vi "Load Clusters from BIN FIles_Core.vi"() -> (1 "System settings":T1={"CONFIG Folder - Relative Path "=path "", "FIFO Depth (# of elements)"=0, "Avoid ALARM/ TRIP in transient regimes?"=FALSE, "Sample Rate [Hz]"=0.0, "Processing interval [s]"=0.0, "Total number of channels to read from FPGA  (auto-calculated)"=0, "# of data to read-DMA (auto-calculated)"=0, "SysLog Interval (s)"=0, "Running Log Folder - Relative Path "=path "Logs/Running_Log", "Reset Log File - Relative Path "=path "Logs/ResetLogs/cRIO_reset.txt", "Error Log File - Relative Path "=path "Logs/Running_Log", "Ring Buffer Size (# Log File Elements)"=86400, "CPU Usage Exceed Limit ()"=98.0, "CPU Usage Exceed Limit Delay (# of iterrations)"=86400, "Free Memory Min Avail.  (%)"=98.0, "Base CoDiS Folder"=path "c:/CoDiS", "Archive Log Folder - Relative Path "=path "Logs/Archive_Log", "Avail. Drive Space Limit to do Archive (%)"=20.0, "Mediator IP address"="10.50.10.1", "Mediator Communication TCP/IP Port"=20, "Used channels (from FPGA) per units -Auto calculated"=[], "# DMA FIFO Fulls File - Relative Path "=path "Logs/ResetLogs/cRIO_reset.txt", "Log Status Parameters in cRIO Ring Buffer"=FALSE, "Channels Input Configuration (has to be defined for all available AI)"=[], "Index to check OL and SC (from FPGA) per units and channels -Auto calculated)"=[], "System not OK? (Auto-calculated)"=FALSE, "System not OK Relay Number (-1 = none, 0,..., MAX)"=-1, "Use normal (T) or inverse (F) relay logic for given relay (size of array equals to number of relays)?"=[], "U32 Relay Output (Auto-calculated)"=0, "cRIO Source"=enum."Not Used", "Check DMA FIFO Full?"=FALSE, "Modbus Settings"={"Modbus Communication Port"=502, "Run as Modbus Server/Slave? (FALSE=Modbus Client/Master)"=FALSE, "Modbus Slave Remote IP Address (if Run as Modbus Server/Slave?=FALSE)"=""}, "Time Synchronization Settings"={"Enable Time Synchronization"=FALSE, "Time Server IP Address (if Enable Time Synchronization=TRUE)"=""}} {"Channels Input Configuration (has to be defined for all available AI)" items=["AC Coupled", "DC Coupled", "IEPE AC Coupled", "Not DSA Channel"]}, 2 "Pan Cluster":T4[](array[typedef]) {"Absolute Minimum Air Gap per Plane"."Absolute AG Minimum Pole Number" format="%.3f"; "Absolute Minimum Air Gap per Plane"."Absolute AG Minimum Value" format="%.3f"; "Magnetic Field Data"."Maximum by Pole Number" format="%.3f"; "Air Gap Data"."Minimum by Pole Number" format="%.3f"; "Orbit(s) - XY"."Orbit XY Graphs (Synthesized from Selected Harmonics and DC)"."?" format="%.3f"; "Orbit(s) - XY"."Orbit XY Graphs (Synthesized from Selected Harmonics and DC)"."?" format="%.3f"; "Orbit(s) - XY"."Orbit XY Graphs (Glided and Averaged on One Revolution)"."?" format="%.3f"; "Orbit(s) - XY"."Orbit XY Graphs (Glided and Averaged on One Revolution)"."?" format="%.3f"; "Orbit(s) - XY"."Orbit XY Graphs (Unaveraged)"."?" format="%.3f"; "Orbit(s) - XY"."Orbit XY Graphs (Unaveraged)"."?" format="%.3f"}, 3 "Wav settings":T7[](array[typedef]) {"Analysis Parameters"."SP2Pmax"."Filter Parameters"."low cutoff freq: fl" format="%0.4f"; "Analysis Parameters"."SP2Pmax"."Filter Parameters"."high cutoff freq: fh" format="%0.2f"; "Analysis Parameters"."LoadAngleDelta"."Multiplication Factor" format="%.1f"; "Analysis Parameters"."LoadAngleDelta"."What harmonic? (for example 24th (48 pole machine))" format="%.1f"; "Analysis Parameters"."Peak2Peak"."Filter Parameters"."low cutoff freq: fl" format="%0.4f"; "Analysis Parameters"."Peak2Peak"."Filter Parameters"."high cutoff freq: fh" format="%0.2f"; "Analysis Parameters"."RMS"."Filter Parameters"."order" format="%0.4f"; "Analysis Parameters"."RMS"."Filter Parameters"."low cutoff freq: fl" format="%0.2f"; "Analysis Parameters"."RMS"."Filter Parameters"."high cutoff freq: fh" format="%0.2f"; "Analysis Parameters"."EqPeak"."Filter Parameters"."low cutoff freq: fl" format="%0.4f"; "Analysis Parameters"."EqPeak"."Filter Parameters"."high cutoff freq: fh" format="%0.2f"; "Analysis Parameters"."Peak"."Filter Parameters"."low cutoff freq: fl" format="%0.4f"; "Analysis Parameters"."Peak"."Filter Parameters"."high cutoff freq: fh" format="%0.2f"; "Analysis Parameters"."snPh"."What harmonic?" format="%.1f"; "Analysis Parameters"."snA"."Multiplication Factor" format="%.1f"; "Analysis Parameters"."snA"."What harmonic?" format="%.1f"; "Analysis Parameters"."Smax"."Filter Parameters"."low cutoff freq: fl" format="%0.4f"; "Analysis Parameters"."Smax"."Filter Parameters"."high cutoff freq: fh" format="%0.2f"; "Analysis Parameters"."RPM"."Signal Threshold" format="%.1f"})   [LabVIEW 2011]
uses:
  CoDiS_Core.llb/Waveforms_cluster_Erraring.ctl
  CoDiS_Core.llb/Unit_names_Erraring.ctl
  CoDiS_Core.llb/Data_sources_Erraring.ctl
  CoDiS_Core.llb/Types_of_signals_Erraring.ctl
  CoDiS_Core.llb/Types_of_analyses_Erraring.ctl
  CoDiS_Core.llb/Analysis_parameters_cluster_Erraring.ctl
  <vilib>/Analysis/3filter.llb/Filter Passband Type.ctl
  CoDiS_Core.llb/Integration_types_Erraring.ctl
  CoDiS_Core.llb/Pan_cluster_Erraring.ctl
  CoDiS_Core.llb/Condition_vector_cluster_Erraring.ctl
  CoDiS_Core.llb/cRIO_system_settings_cluster_Erraring.ctl
  CoDiS_Core.llb/DSA Channels Configuration for Admin_Erraring.ctl
  <vilib>/Analysis/NI_AALBase.lvlib
panel:
  out "error out":errorcluster
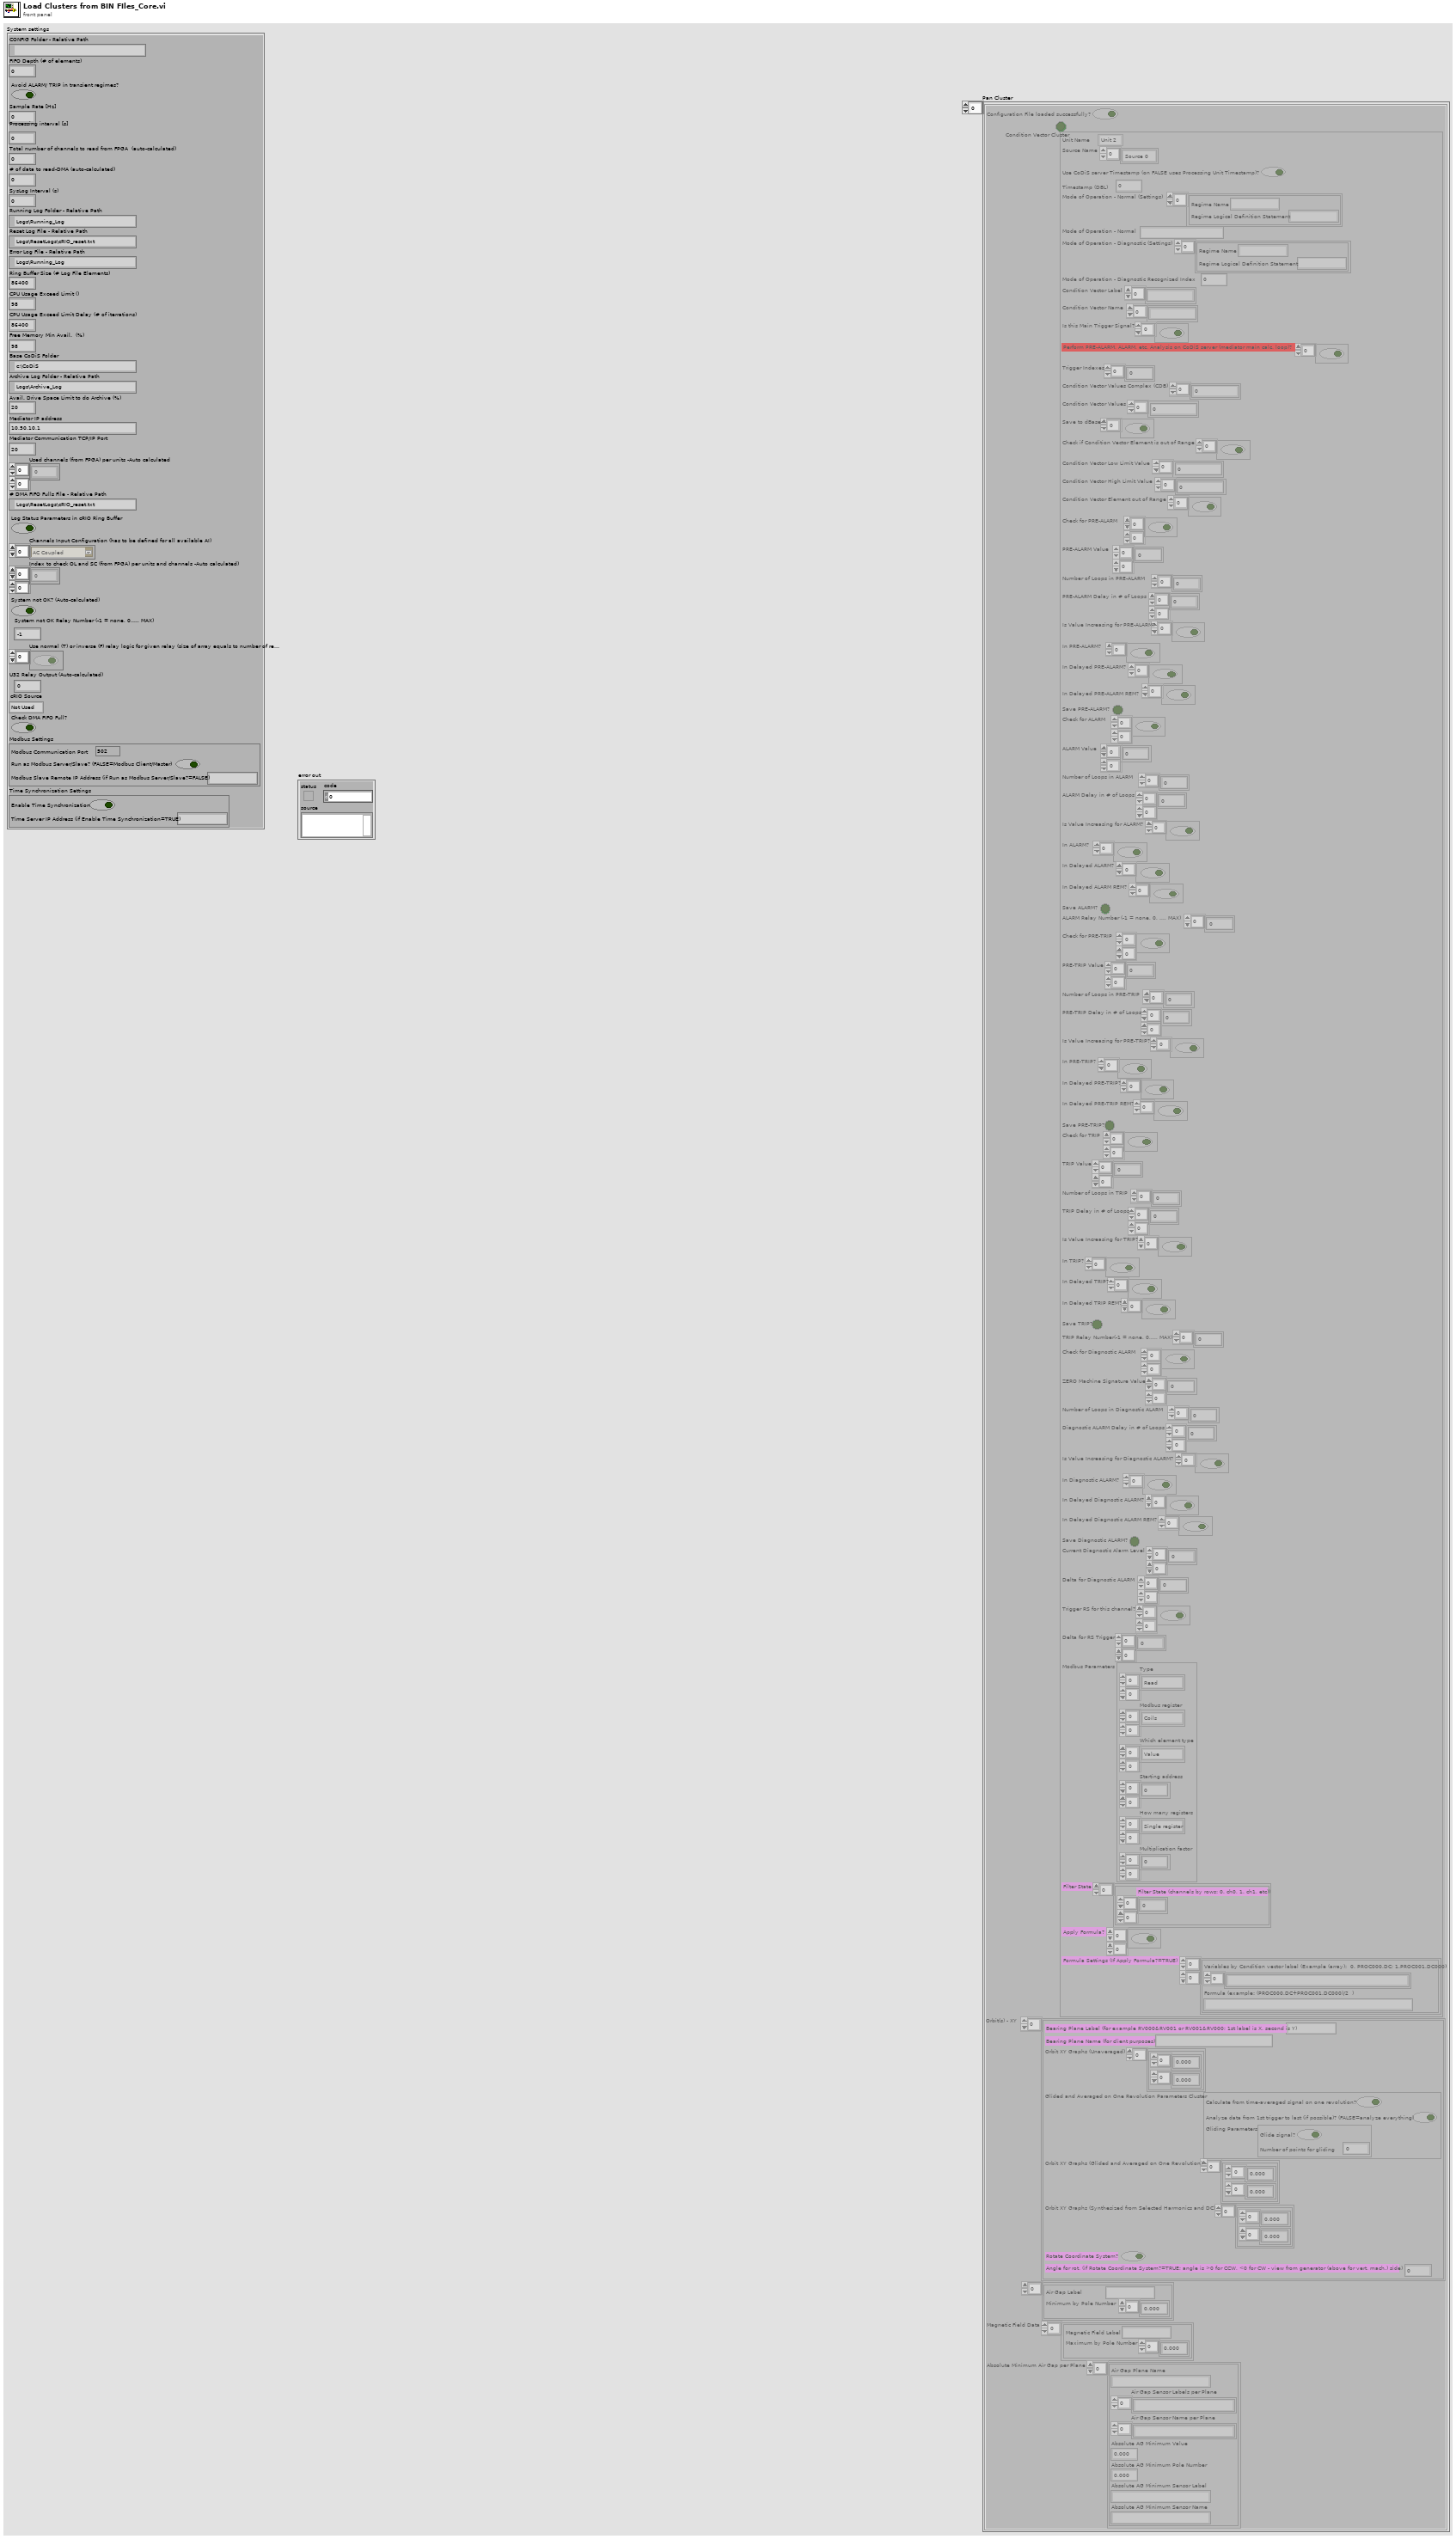
[diagram p1: front panel]
types:
  T1 = typedef "cRIO_system_settings_cluster_Erraring.ctl" = cluster{"CONFIG Folder - Relative Path ":path, "FIFO Depth (# of elements)":u32, "Avoid ALARM/ TRIP in transient regimes?":bool, "Sample Rate [Hz]":sgl, "Processing interval [s]":sgl, "Total number of channels to read from FPGA  (auto-calculated)":u32, "# of data to read-DMA (auto-calculated)":u32, "SysLog Interval (s)":u32, "Running Log Folder - Relative Path ":path, "Reset Log File - Relative Path ":path, "Error Log File - Relative Path ":path, "Ring Buffer Size (# Log File Elements)":u32, "CPU Usage Exceed Limit ()":sgl, "CPU Usage Exceed Limit Delay (# of iterrations)":u32, "Free Memory Min Avail.  (%)":sgl, "Base CoDiS Folder":path, "Archive Log Folder - Relative Path ":path, "Avail. Drive Space Limit to do Archive (%)":sgl, "Mediator IP address":string, "Mediator Communication TCP/IP Port":u16, "Used channels (from FPGA) per units -Auto calculated":i32[][], "# DMA FIFO Fulls File - Relative Path ":path, "Log Status Parameters in cRIO Ring Buffer":bool, "Channels Input Configuration (has to be defined for all available AI)":T2[], "Index to check OL and SC (from FPGA) per units and channels -Auto calculated)":i32[][], "System not OK? (Auto-calculated)":bool, "System not OK Relay Number (-1 = none, 0,..., MAX)":i16, "Use normal (T) or inverse (F) relay logic for given relay (size of array equals to number of relays)?":bool[], "U32 Relay Output (Auto-calculated)":u32, "cRIO Source":T3, "Check DMA FIFO Full?":bool, "Modbus Settings":cluster{"Modbus Communication Port":u16, "Run as Modbus Server/Slave? (FALSE=Modbus Client/Master)":bool, "Modbus Slave Remote IP Address (if Run as Modbus Server/Slave?=FALSE)":string}, "Time Synchronization Settings":cluster{"Enable Time Synchronization":bool, "Time Server IP Address (if Enable Time Synchronization=TRUE)":string}}
  T2 = typedef "DSA Channels Configuration for Admin_Erraring.ctl" = u16
  T3 = typedef "Data_sources_Erraring.ctl" = enum16{"Not Used", "Source 0", "Source 1", "Source 2", "Source 3", "Source 4", "Source 5", "Source 6", "Source 7", "Source 8", "Source 9", "Source 10", "Source 11", "Source 12", "Source 13", "Source 14", "Source 15", "Source 16", "Source 17", "Source 18", "Source 19", "Source 20"}
  T4 = typedef "Pan_cluster_Erraring.ctl" = cluster{"Configuration File loaded successfully?":bool, "Is this new configuration?":bool, "Condition Vector Cluster":T5, "Orbit(s) - XY":cluster{"Bearing Plane Label (for example RV000&RV001 or RV001&RV000; 1st label is X, second is Y)":string, "Bearing Plane Name (for client purposes)":string, "Orbit XY Graphs (Unaveraged)":cluster{sgl[], sgl[]}[], "Glided and Averaged on One Revolution Parameters Cluster":cluster{"Calculate from time-averaged signal on one revolution?":bool, "Analyze data from 1st trigger to last (if possible)? (FALSE=analyze everything)":bool, "Gliding Parameters":cluster{"Glide signal?":bool, "Number of points for gliding":u16}}, "Orbit XY Graphs (Glided and Averaged on One Revolution)":cluster{sgl[], sgl[]}[], "Orbit XY Graphs (Synthesized from Selected Harmonics and DC)":cluster{sgl[], sgl[]}[], "Rotate Coordinate System?":bool, "Angle for rot. (if Rotate Coordinate System?=TRUE; angle is >0 for CCW, <0 for CW - view from generator (above for vert. mach.) side)":sgl}[], "Air Gap Data":cluster{"Air Gap Label":string, "Minimum by Pole Number":sgl[]}[], "Magnetic Field Data":cluster{"Magnetic Field Label":string, "Maximum by Pole Number":sgl[]}[], "Absolute Minimum Air Gap per Plane":cluster{"Air Gap Plane Name":string, "Air Gap Sensor Labels per Plane":string[], "Air Gap Sensor Name per Plane":string[], "Absolute AG Minimum Value":sgl, "Absolute AG Minimum Pole Number":sgl, "Absolute AG Minimum Sensor Label":string, "Absolute AG Minimum Sensor Name":string}[]}
  T5 = typedef "Condition_vector_cluster_Erraring.ctl" = cluster{"Unit Name":T6, "Source Name":T3[], "Use CoDiS server Timestamp (on FALSE uses Processing Unit Timestamp)?":bool, "Timestamp (DBL)":dbl, "Mode of Operation - Normal (Settings)":cluster{"Regime Name":string, "Regime Logical Definition Statement":string}[], "Mode of Operation - Normal":string, "Mode of Operation - Diagnostic (Settings)":cluster{"Regime Name":string, "Regime Logical Definition Statement":string}[], "Mode of Operation - Diagnostic Recognized Index":i16, "Condition Vector Label":string[], "Condition Vector Name":string[], "Is this Main Trigger Signal?":bool[], "Perform PRE-ALARM, ALARM, etc. Analysis on CoDiS server (mediator main calc. loop)?":bool[], "Trigger Indexes":u32[], "Condition Vector Values Complex (CDB)":cdb[], "Condition Vector Values":sgl[], "Save to dBase":bool[], "Check if Condition Vector Element is out of Range":bool[], "Condition Vector Low Limit Value":sgl[], "Condition Vector High Limit Value":sgl[], "Condition Vector Element out of Range":bool[], "Check for PRE-ALARM":bool[][], "PRE-ALARM Value":sgl[][], "Number of Loops in PRE-ALARM":u32[], "PRE-ALARM Delay in # of Loops":u16[][], "Is Value Increasing for PRE-ALARM?":bool[], "In PRE-ALARM?":bool[], "In Delayed PRE-ALARM?":bool[], "In Delayed PRE-ALARM REM?":bool[], "Save PRE-ALARM?":bool, "Check for ALARM":bool[][], "ALARM Value":sgl[][], "Number of Loops in ALARM":u32[], "ALARM Delay in # of Loops":u16[][], "Is Value Increasing for ALARM?":bool[], "In ALARM?":bool[], "In Delayed ALARM?":bool[], "In Delayed ALARM REM?":bool[], "Save ALARM?":bool, "ALARM Relay Number (-1 = none, 0, ..., MAX)":i16[], "Check for PRE-TRIP":bool[][], "PRE-TRIP Value":sgl[][], "Number of Loops in PRE-TRIP":u32[], "PRE-TRIP Delay in # of Loops":u16[][], "Is Value Increasing for PRE-TRIP?":bool[], "In PRE-TRIP?":bool[], "In Delayed PRE-TRIP?":bool[], "In Delayed PRE-TRIP REM?":bool[], "Save PRE-TRIP?":bool, "Check for TRIP":bool[][], "TRIP Value":sgl[][], "Number of Loops in TRIP":u32[], "TRIP Delay in # of Loops":u16[][], "Is Value Increasing for TRIP?":bool[], "In TRIP?":bool[], "In Delayed TRIP?":bool[], "In Delayed TRIP REM?":bool[], "Save TRIP?":bool, "TRIP Relay Number(-1 = none, 0,..., MAX)":i16[], "Check for Diagnostic ALARM":bool[][], "ZERO Machine Signature Value":dbl[][], "Number of Loops in Diagnostic ALARM":u32[], "Diagnostic ALARM Delay in # of Loops":u16[][], "Is Value Increasing for Diagnostic ALARM?":bool[], "In Diagnostic ALARM?":bool[], "In Delayed Diagnostic ALARM?":bool[], "In Delayed Diagnostic ALARM REM?":bool[], "Save Diagnostic ALARM?":bool, "Current Diagnostic Alarm Level":sgl[][], "Delta for Diagnostic ALARM":sgl[][], "Trigger RS for this channel?":bool[][], "Delta for RS Trigger":sgl[][], "Modbus Parameters":cluster{"Type":enum16{"Read", "Write", "None"}[][], "Modbus register":enum16{"Coils", "Discrete Inputs", "Input Registers", "Holding Registers"}[][], "Which element type":enum16{"Value", "Alarm", "Trip"}[][], "Starting address":u16[][], "How many registers":enum16{"Single register", "HI-LO", "LO-HI"}[][], "Multiplication factor":dbl[][]}, "Filter State":cluster{"Filter State (channels by rows: 0. ch0, 1. ch1, etc))":dbl[][]}[], "Apply Formula?":bool[][], "Formula Settings (If Apply Formula?=TRUE)":cluster{"Variables by Condition vector label (Example (array):  0. PROC000.DC; 1.PROC001.DC000)":string[], "Formula (example: (PROC000.DC+PROC001.DC000)/2  )":string}[][]}
  T6 = typedef "Unit_names_Erraring.ctl" = enum16{"Not used", "Unit 1", "Unit 2", "Unit 3", "Unit 4", "Unit 5", "Unit 6", "Unit 7", "Unit 8", "Unit 9"}
  T7 = typedef "Waveforms_cluster_Erraring.ctl" = cluster{"Configuration File loaded successfully? ":bool, "Is this new configuration?":bool, "Unit Name":T6, "Waveform Source":T3[], "Use CoDiS server Timestamp (on FALSE uses Processing Unit Timestamp)?":bool, "Sampling Rate [Hz]":u32[], "Timestamp (DBL)":dbl, "Mode of Operation - Normal":string, "Mode of Operation - Diagnostic":string, "Waveform Physical Channel":u16[], "Waveform Label":string[], "Waveform Name":string[], "Signal Type":cluster{"Signal Type":T8, "# of signal of particular type":u8}[], "Is this Main Trigger Signal?":bool[], "Slope":dbl[], "Intercept":dbl[], "Waveform Values":sgl[][], "Analyse?":bool[], "Save to database?":bool[], "Analyses to Perform":T9[][], "Perform this analysis on a CoDiS server?":bool[][], "General Parameters":cluster{"Number of Poles":u8, "Grid Frequency":sgl}, "Analysis Parameters":T10[][], "Save now to dBase?":bool, "Waveform Length for Saving [s]":u16, "Pretrigger Length when Saving Waveform [s]":u16, "Next Timestamp to autosave at (DBL)":dbl, "Description of Waveforms Events":string, "Event Type":string, "Save next RS event entirely? (on FALSE uses How many basic (acquisition) blocks of data (loops) to save?":bool, "Regime Name for which to save next RS event entirely":string, "Integration type":T12[], "Channel not OK?":bool[], "Channel Not OK?  Relay Number (-1 = none, 0, ..., MAX)":i16[], "Array of FPGA Filter Parameters":cluster{"Filter signal?":bool, "filter type":T11, "high cutoff freq: fh":dbl, "low cutoff freq: fl":dbl, "order":i32}[][], "Pre-Alarm Delay in Number of Loops ":u16, "Pre-Trip Delay in Number of Loops ":u16}
  T8 = typedef "Types_of_signals_Erraring.ctl" = enum16{"Not Used", "Trigger (TRG???)", "Relative Vibrations (RV???)", "Absolute Vibrations (AV???)", "Air Gap (AG???)", "Magnetic Field (MX???)", "Voltage (VOL???)", "Current (CURR???)", "Process (PROC???)", "Cavitation (CAV???)", "Non Standard (NONST???)", "Axial Displacement (AXD???)", "Absolute Vibrations Stator Core (AVSC???)"}
  T9 = typedef "Types_of_analyses_Erraring.ctl" = enum16{"Exit Analysis Loop", "Do Nothing", "RPM", "Smax", "SP2Pmax", "snA", "snPh", "Rest", "Peak", "EqPeak", "Peak2Peak", "RMS", "DC", "DC from Extrema", "Min Value", "Max Value", "Min Value by Pole", "Max Value by Pole", "Max Diff by Pole", "Max Diff Pole Number", "Min from Extrema", "Max from Extrema", "Active Power from DFT", "Active Power by Integration", "Reactive Power from DFT", "Reactive Power by Integration", "Apparent Power", "Ampl@Freq", "Phase Difference", "Load Angle Delta", "THD", "Signal Frequency", "Eta", "Non standard (CoDiS server - manual) 0", "Non standard (CoDiS server - manual) 1", "Non standard (CoDiS server - manual) 2", "Non standard (CoDiS server - manual) 3", "Non standard (CoDiS server - manual) 4", "Non standard (CoDiS server - manual) 5", "Non standard (CoDiS server - manual) 6", "Non standard (CoDiS server - manual) 7", "Non standard (CoDiS server - manual) 8", "Non standard (CoDiS server - manual) 9", "Non standard (CoDiS server - manual) 10", "Non standard (CoDiS server - manual) 11", "Non standard (CoDiS server - manual) 12", "Non standard (CoDiS server - manual) 13", "Non standard (CoDiS server - manual) 14", "Non standard (CoDiS server - manual) 15", "Non standard (CoDiS server - manual) 16", "Non standard (CoDiS server - manual) 17", "Non standard (CoDiS server - manual) 18", "Non standard (CoDiS server - manual) 19", "CosFi", "Total THD", "Crest Factor"}
  T10 = typedef "Analysis_parameters_cluster_Erraring.ctl" = cluster{"DC":cluster{"Analyze data from 1st trigger to last (if possible)? (FALSE=analyze everything)":bool}, "DCExtrema":cluster{"Calculate DC from all Pole Values":bool, "Poles to use in DC calculation (if Calculate DC from all Pole Values is FALSE)":u8[], "Condition Vector Label begin Part (MinPole or MaxPole)":string, "Addition to Condition Vector Label (example: 000)":string}, "RPM":cluster{"Signal Threshold":sgl, "Pulse Width (should be >= 2 depending on signal noise)":i32, "Trigger on rising edge? (FALSE=trigger on falling)":bool}, "Smax":cluster{"Combine with which Waveform Label? (for example: RV001)":string, "Calculate from time-averaged signal on one revolution?":bool, "Analyze data from 1st trigger to last (if possible)? (FALSE=analyze everything)":bool, "Filter Parameters":cluster{"Filter signal?":bool, "filter type":T11, "high cutoff freq: fh":dbl, "low cutoff freq: fl":dbl, "order":i32, "Process as ring-buffer signal?":bool}, "Gliding Parameters":cluster{"Glide signal?":bool, "Number of points for gliding":u16}, "Average all calculated values for Smax - if present (each revolution)? (FALSE=take absolute maximum)":bool, "Addition to Condition Vector Label (example: 000)":string}, "SP2Pmax":cluster{"Combine with which Waveform Label? (for example: RV001)":string, "Calculate from time-averaged signal on one revolution?":bool, "Analyze data from 1st trigger to last (if possible)? (FALSE=analyze everything)":bool, "Filter Parameters":cluster{"Filter signal?":bool, "filter type":T11, "high cutoff freq: fh":dbl, "low cutoff freq: fl":dbl, "order":i32, "Process as ring-buffer signal?":bool}, "Gliding Parameters":cluster{"Glide signal?":bool, "Number of points for gliding":u16}, "Average all calculated values for SP2Pmax - if present (each revolution)? (FALSE=take absolute maximum)":bool, "Addition to Condition Vector Label (example: 000)":string}, "snA":cluster{"What harmonic?":sgl, "Calculate Amplitude (TRUE) or RMS (FALSE)?":bool, "Multiplication Factor":sgl, "Calculate Amplitude for Air Gap type signals? (from MinPole Values)":bool}, "snPh":cluster{"What harmonic?":sgl}, "Peak":cluster{"Calculate from time-averaged signal (one-revolution)?":bool, "Analyze data from 1st trigger to last (if possible)? (FALSE=analyze everything)":bool, "Filter Parameters":cluster{"Filter signal?":bool, "filter type":T11, "high cutoff freq: fh":dbl, "low cutoff freq: fl":dbl, "order":i32, "Process as ring-buffer signal?":bool}, "Gliding Parameters":cluster{"Glide signal?":bool, "Number of points for gliding":u16}, "Average all calculated values for Peak - if present (each revolution)? (FALSE=take absolute maximum)":bool, "Addition to Condition Vector Label (example: 000)":string}, "Peak2Peak":cluster{"Calculate from time-averaged signal (one-revolution)?":bool, "Analyze data from 1st trigger to last (if possible)? (FALSE=analyze everything)":bool, "Gliding Parameters":cluster{"Glide signal?":bool, "Number of points for gliding":u16}, "Filter Parameters":cluster{"Filter signal?":bool, "filter type":T11, "high cutoff freq: fh":dbl, "low cutoff freq: fl":dbl, "order":i32, "Process as ring-buffer signal?":bool}, "Average all calculated values for Peak2Peak - if present (each revolution)? (FALSE=take absolute maximum)":bool, "Addition to Condition Vector Label (example: 000)":string}, "EqPeak":cluster{"Calculate from time-averaged signal (one-revolution)?":bool, "Analyze data from 1st trigger to last (if possible)? (FALSE=analyze everything)":bool, "Average all calculated values for EqPeak - if present (each revolution)? (FALSE=take absolute maximum)":bool, "Filter Parameters":cluster{"Filter signal?":bool, "filter type":T11, "high cutoff freq: fh":dbl, "low cutoff freq: fl":dbl, "order":i32, "Process as ring-buffer signal?":bool}, "Which Condition Vector Label addition to use for RMS (example: 001)":string, "Addition to Condition Vector Label (example: 000)":string}, "RMS":cluster{"Calculate from time-averaged signal (one-revolution)?":bool, "Analyze data from 1st trigger to last (if possible)? (FALSE=analyze everything)":bool, "Subtract DC before RMS calculation?":bool, "Filter Parameters":cluster{"Filter signal?":bool, "filter type":T11, "high cutoff freq: fh":dbl, "low cutoff freq: fl":dbl, "order":i32, "Process as ring-buffer signal?":bool}, "Gliding Parameters":cluster{"Glide signal?":bool, "Number of points for gliding":u16}, "Average all calculated values for RMS - if present (each revolution)? (FALSE=take absolute maximum)":bool, "Addition to Condition Vector Label (example: 000)":string}, "Rest":cluster{"Calculate from all calculated harmonics?":bool, "Condition Vector Label to use for substraction (if Calculate from all calculated harmonics?=FALSE)":string[], "Calculate by subtracting from EqPeak Value? (FALSE=calculate by subtracting from RMS Value)":bool, "Which Condition Vector Label addition to use for EqPeak (example: 001)":string, "Addition to Condition Vector Label (example: 000)":string}, "MinByPole":cluster{"First Pole Number after Trigger (indexes correspond to Normal regime settings)":u8[], "Are Pole Numbers in ascending order in time?  (indexes correspond to Normal regime settings)":bool[], "Average all calculated values for that Pole? (FALSE=take absolute minimum)":bool, "Coerce Upper Limit":sgl, "Compensate 1st harmonic in waveform?":bool}, "MinExtrema":cluster{"Calculate Min Extrema from all Pole Values":bool, "Poles to use in Min Extrema calculation (if Calculate Min Extrema from all Pole Values is FALSE)":u8[], "Condition Vector Label begin Part (MinPole or MaxPole)":string}, "MaxByPole":cluster{"First Pole Number after Trigger (indexes correspond to Normal regime settings)":u8[], "Are Pole Numbers in ascending order in time? (indexes correspond to Normal regime settings)":bool[], "Average all calculated values for that Pole? (FALSE=take absolute maximum)":bool, "Calculate with abs(Signal)?":bool, "Subtract DC before calculation?":bool, "Coerce Lower Limit":sgl}, "MaxExtrema":cluster{"Calculate Max Extrema from all Pole Values":bool, "Poles to use in Max Extrema calculation (if Calculate Max Extrema from all Pole Values is FALSE)":u8[], "Condition Vector Label begin Part (MinPole or MaxPole)":string}, "MaxDiffByPole":cluster{"First Pole Number after Trigger (indexes correspond to Normal regime settings)":u8[], "Are Pole Numbers in ascending order in time? (indexes correspond to Normal regime settings)":bool[], "Condition Vector Label begin Part (MinPole or MaxPole)":string}, "Min":cluster{"Analyze data from 1st trigger to last (if possible)? (FALSE=analyze everything)":bool, "Calculate from time-averaged signal on one revolution?":bool, "Gliding Parameters":cluster{"Glide signal?":bool, "Number of points for gliding":u16}, "Average all calculated values for Min - if present (each revolution)? (FALSE=take absolute maximum)":bool}, "Max":cluster{"Analyze data from 1st trigger to last (if possible)? (FALSE=analyze everything)":bool, "Calculate from time-averaged signal on one revolution?":bool, "Gliding Parameters":cluster{"Glide signal?":bool, "Number of points for gliding":u16}, "Average all calculated values for Max - if present (each revolution)? (FALSE=take absolute maximum)":bool}, "ActivePower":cluster{"Calculate from Phase Voltages and Currents?":bool, "Phase Voltage Condition Vector Label (R, S, T) (for example: VOL000.s24.00A, VOL001.s24.00A, VOL002.s24.00A)":string[], "Phase Current Condition Vector Label (R, S, T) (for example: CURR000.s24.00A, CURR001.s24.00A, CURR002.s24.00A)":string[]}, "ReactivePower":cluster{"Calculate from Phase Voltages and Currents?":bool, "Phase Voltage Condition Vector Label (R, S, T) (for example: VOL000.s24.00A, VOL001.s24.00A, VOL002.s24.00A)":string[], "Phase Current Condition Vector Label (R, S, T) (for example: CURR000.s24.00A, CURR001.s24.00A, CURR002.s24.00A)":string[]}, "LoadAngleDelta":cluster{"What harmonic? (for example 24th (48 pole machine))":sgl, "Delta0":sgl, "Which Voltage Waveform Label? (for example: VOL000)":string, "Combine (multiply) with which Air Gap Waveform Label? (for example: AG000)":string, "Multiplication Factor":sgl}, "ActivePowerByIntegration":cluster{"Phase Voltage Waveform Labels (R,S,T)":string[], "Phase Current Waveform Labels (R,S,T)":string[], "Analyze data from 1st trigger to last (if possible)? (FALSE=analyze everything)":bool}, "RectivePowerByIntegration":cluster{"Phase Voltage Waveform Vector Labels (R,S,T)":string[], "Phase Current Waveform Labels (R,S,T)":string[], "System Electric Frequency [Hz]":sgl, "Analyze data from 1st trigger to last (if possible)? (FALSE=analyze everything)":bool}, "Ampl@Freq":cluster{"Frequency [Hz]":sgl, "Calculate Amplitude? (FALSE=calculate RMS)":bool}, "PhaseDifference":cluster{"Combine with which Waveform Label?":string}, "CosFi":cluster{"Voltage Waveform Labels (R,S,T)":string[], "Current Waveform Labels (R,S,T)":string[]}, "Total THD":cluster{"THD Condition Vector Label (R, S, T) (for example: VOL000.THD, VOL001.THD, VOL002.THD)":string[]}, "Crest Factor":cluster{"Addition to Condition Vector Label (example: 000)":string, "Which Condition Vector Label addition to use for Peak (example: 001)":string, "Which Condition Vector Label addition to use for RMS (example: 001)":string}}
  T11 = typedef "NI_AALBase.lvlib/Filter Passband Type.ctl" = enum32{"Lowpass", "Highpass", "Bandpass", "Bandstop"}
  T12 = typedef "Integration_types_Erraring.ctl" = enum16{"Do not integrate", "Integrate once", "Integrate twice"}
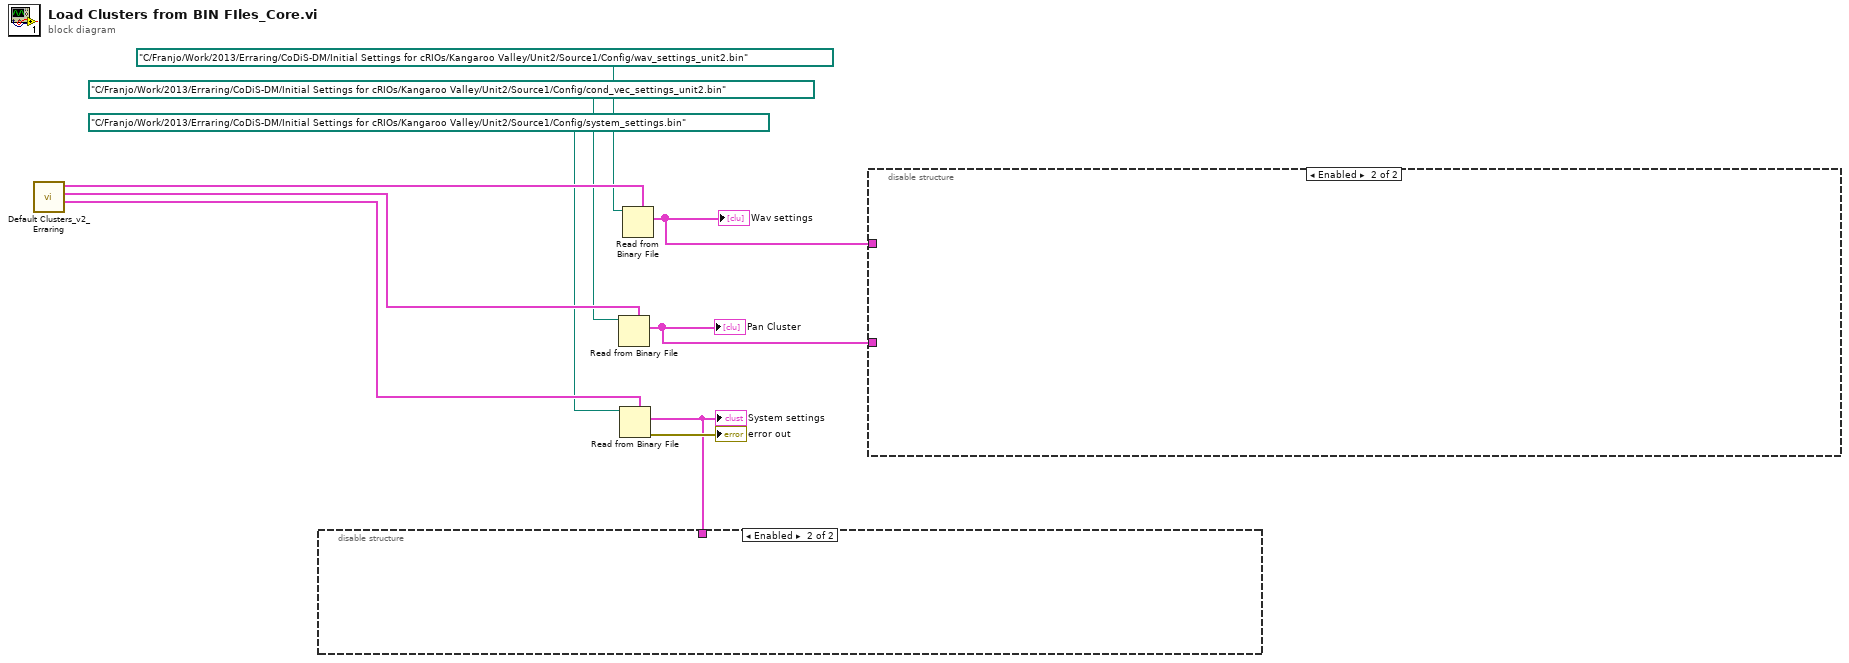
[diagram p0: block diagram]
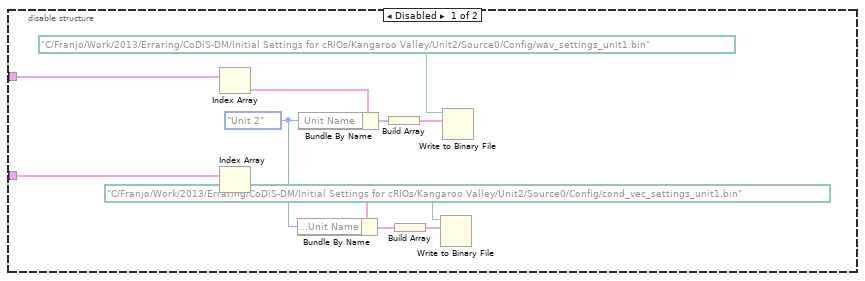
[diagram p2: hidden frame]
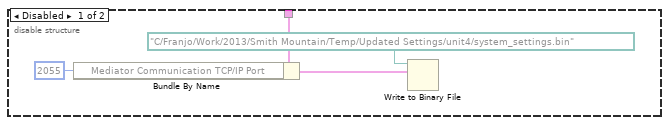
[diagram p3: hidden frame]
diagram:
  n1 = call "Default Clusters_v2_Erraring.vi"() -> ("cRIO System Settings Cluster OUT"=w8:T1, "1D array of Pan Cluster OUT"=w9:T4[], "1D array of Waveform Cluster OUT"=w10:T7[])  [unwired: 8 in, 1 out]
  n2 = Read from Binary File(5:w9, 11:path "C:/Franjo/Work/2013/Erraring/CoDiS-DM/Initial Settings for cRIOs/Kangaroo Valley/Unit2/Source1/Config/cond_vec_settings_unit2.bin" ("file (use dialog)")) -> (2:w2:T4[])  [unwired: 4 in, 3 out]
  "Pan Cluster" <- w2
  n3 = Read from Binary File(5:w8, 11:path "C:/Franjo/Work/2013/Erraring/CoDiS-DM/Initial Settings for cRIOs/Kangaroo Valley/Unit2/Source1/Config/system_settings.bin" ("file (use dialog)")) -> (0:→"error out":errorcluster, 2:w3:T1)  [unwired: 4 in, 2 out]
  "System settings" <- w3
  n4 = disable-structure shown="Enabled" {
    disable-tunnel: w3 -> [w14 _]
    frame Disabled {
      n5 = Bundle By Name(cluster=w14, "Mediator Communication TCP/IP Port"=u16 2055) -> (w12:T1)
      n6 = Write to Binary File(file (use dialog)=path "C:/Franjo/Work/2013/Smith Mountain/Temp/Updated Settings/unit4/system_settings.bin", data=w12) -> ()  [unwired: 4 in, 3 out]
    }
    frame Enabled {
    }
  }
  n7 = Read from Binary File(5:w10, 11:path "C:/Franjo/Work/2013/Erraring/CoDiS-DM/Initial Settings for cRIOs/Kangaroo Valley/Unit2/Source1/Config/wav_settings_unit2.bin" ("file (use dialog)")) -> (2:w1:T7[])  [unwired: 4 in, 3 out]
  "Wav settings" <- w1
  n8 = disable-structure shown="Enabled" {
    disable-tunnel: w1 -> [w25 _]
    disable-tunnel: w2 -> [w24 _]
    frame Disabled {
      w21 = Unit_names_Erraring."Unit 2" ("Unit Name")
      n9 = Index Array(array=w25) -> (element=w23:T7)  [unwired: 1 in]
      n10 = Index Array(array=w24) -> (element=w22:T4)  [unwired: 1 in]
      n11 = Bundle By Name(cluster=w22, "Condition Vector Cluster.Unit Name"=w21) -> (w20:T4)
      n12 = Bundle By Name(cluster=w23, "Unit Name"=w21) -> (w19:T7)
      n13 = Build Array(w19) -> (w18:T7[])
      n14 = Build Array(w20) -> (w17:T4[])
      n15 = Write to Binary File(file (use dialog)=path "C:/Franjo/Work/2013/Erraring/CoDiS-DM/Initial Settings for cRIOs/Kangaroo Valley/Unit2/Source0/Config/cond_vec_settings_unit1.bin", data=w17) -> ()  [unwired: 4 in, 3 out]
      n16 = Write to Binary File(file (use dialog)=path "C:/Franjo/Work/2013/Erraring/CoDiS-DM/Initial Settings for cRIOs/Kangaroo Valley/Unit2/Source0/Config/wav_settings_unit1.bin", data=w18) -> ()  [unwired: 4 in, 3 out]
    }
    frame Enabled {
    }
  }
